vi "Motion_Load Cartridge.vi"(8 "error in":errorcluster, 10 "action":enum16{"Goto Connect", "Goto Load"}(ring)=enum."Goto Load", 11 "TCP address:port":string="192.168.0.3:502") -> (0 "error out":errorcluster, 2 "elapsed time":dbl[unit]=nan format="%.1f")   [LabVIEW 2010]
doc: "This function commands the test set linear actuators to move the test cartridge intothe load or connected positions.\n\nA stopwatch popup is displayed while the cartridge moves into the destination position."
uses:
  Motion_Coils Typedef.ctl
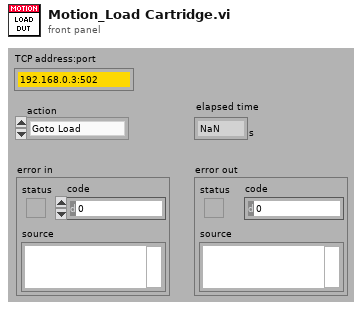
[diagram p1: front panel]
types:
  T1 = typedef "Motion_Coils Typedef.ctl" = u16
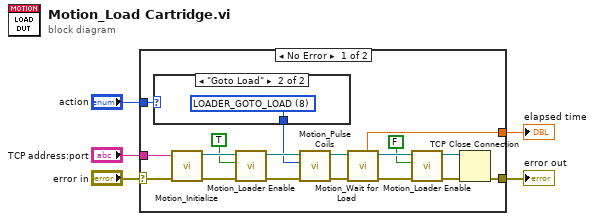
[diagram p0: block diagram]
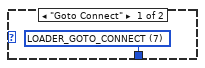
[diagram p2: hidden frame]
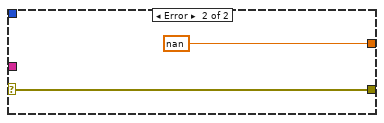
[diagram p3: hidden frame]
diagram:
  n1 = case shown="No Error" "error in" {
    selector: "error in" -> [w19 w27]
    tunnel: [w23 w27] -> w5
    tunnel: "TCP address:port" -> [w18 _]
    tunnel: "action" -> [w12 _]
    tunnel: [w20 dbl[unit] nan ("elapsed time")] -> w1
    frame No Error {
      n2 = case shown="\"Goto Load\"" w12 {
        tunnel: [w24 w25] -> w11
        frame "Goto Connect" {
          w24 = T1 7 items=["GANTRY_ALARM_CLEAR", "GANTRY_ENABLE", "GANTRY_HOME", "GANTRY_GOTO", "LOADER_HOME", "LOADER_ALARM_CLEAR", "LOADER_ENABLE", "LOADER_GOTO_CONNECT", "LOADER_GOTO_LOAD", "LOADER_STOP"] ("Pulse Coil")
        }
        frame "Goto Load" {
          w25 = T1 8 items=["GANTRY_ALARM_CLEAR", "GANTRY_ENABLE", "GANTRY_HOME", "GANTRY_GOTO", "LOADER_HOME", "LOADER_ALARM_CLEAR", "LOADER_ENABLE", "LOADER_GOTO_CONNECT", "LOADER_GOTO_LOAD", "LOADER_STOP"] ("Pulse Coil")
        }
      }
      n3 = call "Motion_Initialize.vi"("error in"=w19, "TCP address:port (192.168.0.3:502)"=w18) -> ("error out"=w15:errorcluster, "connection ID"=w17:refnum<k5>)  [unwired: 8 in]
      n4 = call "Motion_Loader Enable.vi"("error in (no error)"=w15, "Enable? (T)"=TRUE, "TCP Connection Refnum in"=w17) -> ("error out"=w14:errorcluster, "TCP Connection Refnum (dup)"=w16:refnum<k5>)  [unwired: 7 in]
      n5 = call "Motion_Pulse Coils.vi"("error in"=w14, "Pulse Coil"=w11, "TCP refnum"=w16) -> ("error out"=w22:errorcluster, "TCP refnum dup"=w21:refnum<k5>)  [unwired: 7 in]
      n6 = call "Motion_Wait for Load.vi"("error in"=w22, "TCP refnum"=w21) -> ("error out"=w7:errorcluster, "TCP refnum dup"=w10:refnum<k5>, "elapsed time"=w20:dbl[unit])  [unwired: 3 in, 4 out]
      n7 = call "Motion_Loader Enable.vi"("error in (no error)"=w7, "Enable? (T)"=FALSE, "TCP Connection Refnum in"=w10) -> ("error out"=w8:errorcluster, "TCP Connection Refnum (dup)"=w9:refnum<k5>)  [unwired: 7 in]
      n8 = TCP Close Connection(connection ID=w9, error in (no error)=w8) -> (error out=w23:errorcluster)  [unwired: 1 in, 1 out]
    }
    frame Error {
    }
  }
  "error out" <- w5
  "elapsed time" <- w1
